vi "ObjectRegistration.vi"(6 "Min Size":i32=40, 7 "Threshold":i32=30, 8 "error in (no error)":errorcluster, 10 "Roy":T1, 11 "Rob":T1) -> (0 "error out":errorcluster, 1 "Alignment quality":dbl, 2 "y displacement":dbl, 3 "x displacement":dbl)   [LabVIEW 2012]
uses:
  <vilib>/vision/Image Controls.llb/IMAQ Image.ctl
panel:
  out "Roy 2":T1(plugin-control)
  out "Roy":T1(plugin-control)
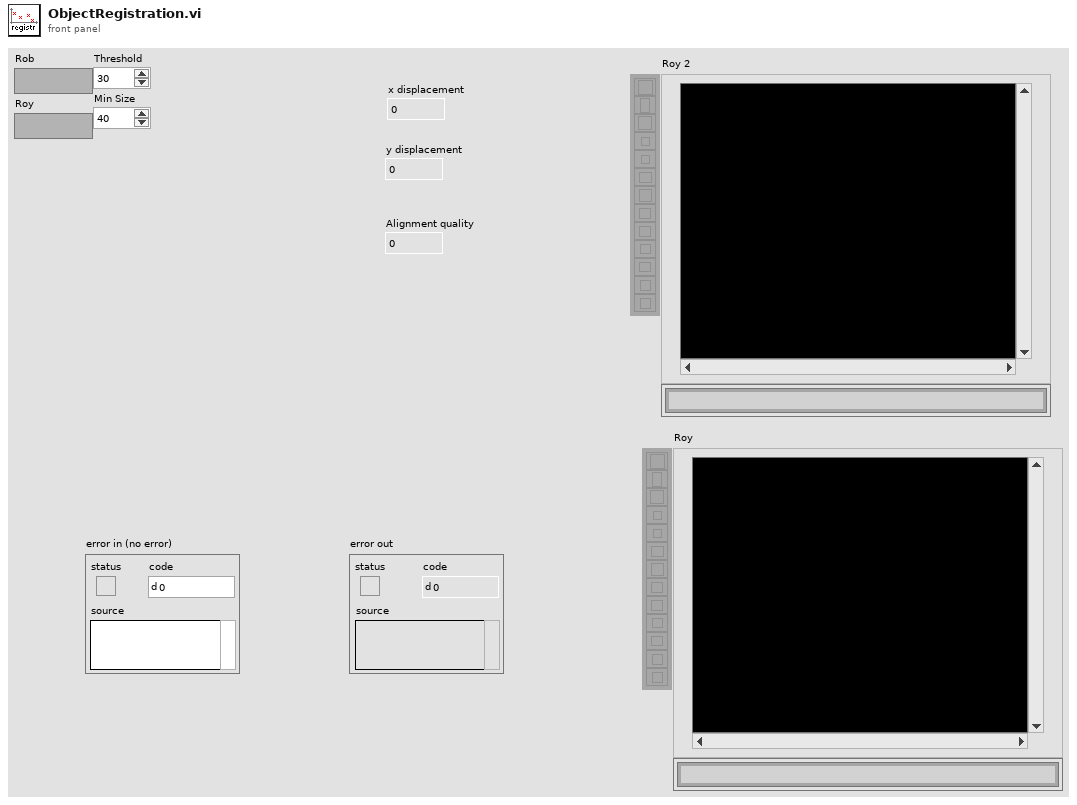
[diagram p1: front panel]
types:
  T1 = typedef "IMAQ Image.ctl" = refnum<image>
  T2 = cluster{"Objects":u16, "Threshold":i32, "Reject Border":bool, "Fill Holes":bool, "Min Object Size":bool, "Min Size":i32, "Max Object Size":bool, "Max Size":i32, "Show Search Area":bool, "Show Center":bool, "Show Bounding Box":bool}
  T3 = cluster{"Object Center":cluster{"X":sgl, "Y":sgl}, "Bounding Box":cluster{"X Left":i32, "Y Top":i32, "X Right":i32, "Y Bottom":i32}, "Area":sgl, "Orientation":sgl, "Aspect Ratio":sgl, "Nb Holes":i32}[]
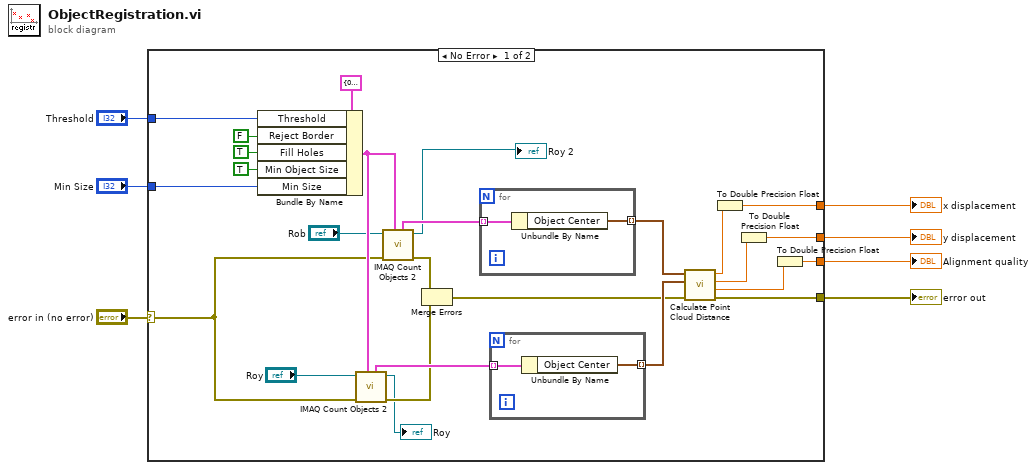
[diagram p0: block diagram]
diagram:
  n1 = case shown="No Error" "error in (no error)" {
    selector: "error in (no error)" -> [w19 w38]
    tunnel: [w18 w38] -> w6
    tunnel: [w14 _] -> w5
    tunnel: [w13 _] -> w4
    tunnel: [w12 _] -> w3
    tunnel: "Threshold" -> [w9 _]
    tunnel: "Min Size" -> [w8 _]
    frame No Error {
      n2 = Bundle By Name(cluster=T2 {"Objects"=0, "Threshold"=128, "Reject Border"=FALSE, "Fill Holes"=FALSE, "Min Object Size"=FALSE, "Min Size"=3, "Max Object Size"=FALSE, "Max Size"=100, "Show Search Area"=FALSE, "Show Center"=TRUE, "Show Bounding Box"=TRUE} ("Settings"), "Threshold"=w9, "Reject Border"=FALSE, "Fill Holes"=TRUE, "Min Object Size"=TRUE, "Min Size"=w8) -> (w29:T2)
      n3 = call "IMAQ Count Objects 2"("Settings"=w29, "error in (no error)"=w19, "Image"="Roy") -> ("error out"=w22:errorcluster, "Image Out"=→"Roy":T1, "Objects"=w27:T3)  [unwired: 4 in, 2 out]
      n4 = call "IMAQ Count Objects 2"("Settings"=w29, "error in (no error)"=w19, "Image"="Rob") -> ("error out"=w21:errorcluster, "Image Out"=→"Roy 2":T1, "Objects"=w28:T3)  [unwired: 4 in, 2 out]
      n5 = Merge Errors(w21, w22) -> (w20:errorcluster)
      n6 = for {
        tunnel: w28 -> [w37] mode=indexing
        tunnel: [w36] -> w26 mode=indexing
        n7 = Unbundle By Name(w37) -> ("Object Center"=w36:cluster{"X":sgl, "Y":sgl})
      }
      n8 = for {
        tunnel: w27 -> [w35] mode=indexing
        tunnel: [w34] -> w25 mode=indexing
        n9 = Unbundle By Name(w35) -> ("Object Center"=w34:cluster{"X":sgl, "Y":sgl})
      }
      n10 = call "Calculate Point Cloud Distance.vi"("error in (no error)"=w20, "Moving point cloud"=w25, "Fixed point cloud"=w26) -> ("error out"=w18:errorcluster, "Alignment quality"=w17:sgl, "y displacement"=w16:sgl, "x displacement"=w15:sgl)  [unwired: 5 in]
      n11 = To Double Precision Float(number=w15) -> (double precision float=w12:dbl)
      n12 = To Double Precision Float(number=w16) -> (double precision float=w13:dbl)
      n13 = To Double Precision Float(number=w17) -> (double precision float=w14:dbl)
    }
    frame Error {
    }
  }
  "x displacement" <- w3
  "y displacement" <- w4
  "Alignment quality" <- w5
  "error out" <- w6
